vi "Download_Save.vi"(8 "error in (no error)":errorcluster, 10 "Data Feed":string, 11 "DataCluster":T1) -> (0 "error out":errorcluster)   [LabVIEW 2020]
uses:
  DataCluster.ctl
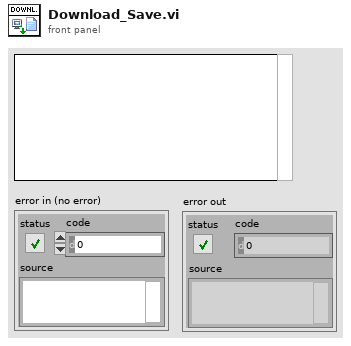
[diagram p1: front panel]
types:
  T1 = typedef "DataCluster.ctl" = cluster{"Core":cluster{"Current VI Reference":refnum<vi>, "Close Panel on Exit?":bool, "Exit":bool}, "Connections":cluster{"Arduino":cluster{"VISA":refnum<visa-resource-name>, "Data Feed":string, "Connected":bool}, "Ready":bool}, "Files":cluster{"Path":path, "Filename":string, "File List":i32, "Buffer":cluster{"Buffer":refnum<queue>, "Size":i32}, "Downloading":bool}}
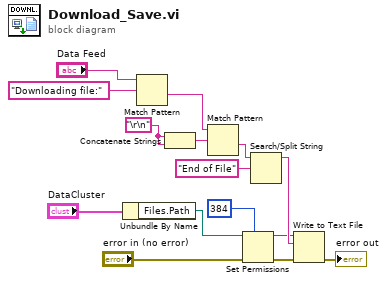
[diagram p0: block diagram]
diagram:
  w12 = "\r\n"
  n1 = Unbundle By Name("DataCluster") -> ("Files.Path"=w1:path)
  n2 = Match Pattern(string="Data Feed", regular expression="Downloading file:") -> (after substring=w13:string)  [unwired: 1 in, 3 out]
  n3 = Concatenate Strings(w12, w12) -> (w14:string)
  n4 = Match Pattern(string=w13, regular expression=w14) -> (after substring=w15:string)  [unwired: 1 in, 3 out]
  n5 = Set Permissions(7:i16 384 ("permissions"), 8:"error in (no error)", 11:w1) -> (0:w4:errorcluster, 3:w3:path)  [unwired: 2 in]
  n6 = Search/Split String(string=w15, search string/char (-)="End of File") -> (substring before match=w7:string)  [unwired: 1 in, 2 out]
  n7 = Write to Text File(file (use dialog)=w3, text=w7, error in=w4) -> (error out=→"error out":errorcluster)  [unwired: 1 in, 2 out]
